vi "Write frozen.vi"(8 "error in (no error)":errorcluster, 10 "frozen":bool, 11 "PongBall in":refnum<class "PongBall.lvclass">) -> (0 "error out":errorcluster, 3 "PongBall out":refnum<class "PongBall.lvclass">)   [LabVIEW 2019, in "RT_Game.lvlib" / "PongBall.lvclass"]
uses:
  PongBall.lvclass
  PongBall.lvclass/PongBall.ctl
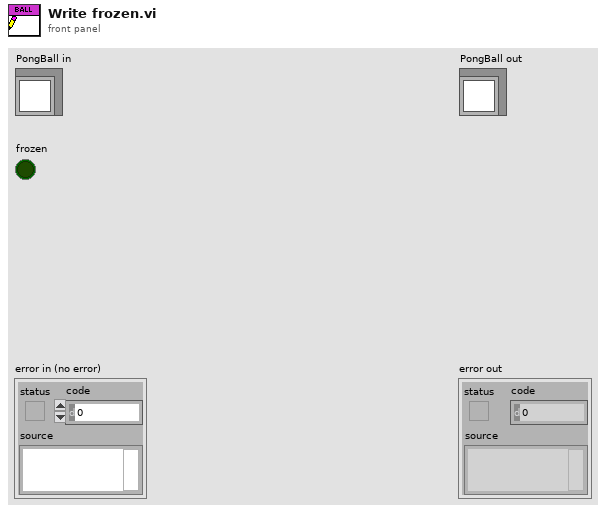
[diagram p1: front panel]
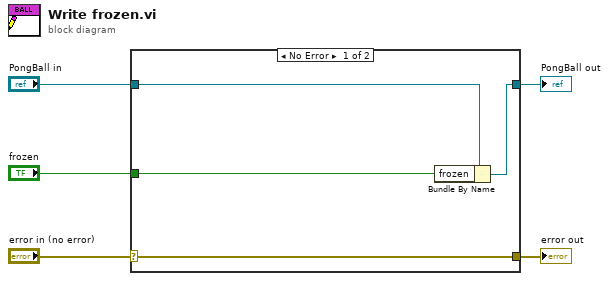
[diagram p0: block diagram]
diagram:
  n1 = case shown="No Error" "error in (no error)" {
    selector: "error in (no error)" -> [w9 w10]
    tunnel: [w9 w10] -> w4
    tunnel: [w7 w11] -> w2
    tunnel: "PongBall in" -> [w8 w11]
    tunnel: "frozen" -> [w6 _]
    frame No Error {
      n2 = Bundle By Name(cluster=w8, "frozen"=w6) -> (w7:refnum<class "PongBall.lvclass">)
    }
    frame Error {
    }
  }
  "error out" <- w4
  "PongBall out" <- w2
